vi "ClassList Playground.vi"() -> ()   [LabVIEW 2019]
uses:
  Classes/Subpanel/Edit/Edit/Edit.lvclass
  Classes/Settings/Setting Database/Setting Database.lvclass
  C:/Program Files (x86)/National Instruments/LabVIEW 2019/vi.lib/JKI/JKI SMO/SMO/SMO.lvclass
  Classes/Settings/Setting Database/Typedefs/PrivateEvents--Setting Database.Refresh.ctl
  Classes/Settings/Setting Database/Typedefs/PrivateEvents--Setting Database.SetActivePath.ctl
  Classes/Settings/Setting Database/Typedefs/PrivateEvents--Setting Database.Add To Group.ctl
  Classes/Settings/Setting Database/Typedefs/PrivateEvents--Setting Database.SetActiveRectangle.ctl
  Classes/Subpanel/Manager/Subpanel.Edit.lvclass
  C:/Users/Albro/Documents/GitHub/AFM-Lithography/lvsrc/Classes/Subpanel/Subpanel.lvclass
  Classes/Subpanel/Edit/Edit.Path/Edit.Path.lvclass
  <vilib>/JKI/JKI SMO/SMO/SMO.lvclass
  Classes/Subpanel/Subpanel.lvclass
  C:/Users/Albro/Documents/GitHub/AFM-Lithography/lvsrc/Classes/Subpanel/Edit/Edit/Edit.lvclass
panel:
  out "Array":T1(array[cluster])
  in  "Key":string="p"
  out "key not found?":bool
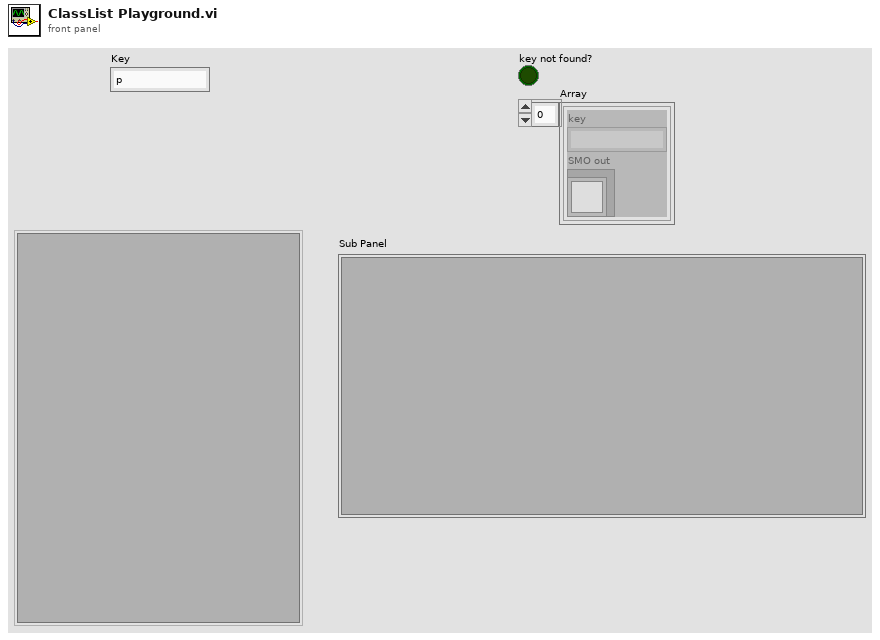
[diagram p1: front panel]
types:
  T1 = cluster{"key":string, "SMO out":refnum<class "Edit.lvclass">}[]
  T2 = typedef "Setting Database.lvclass/PrivateEvents--Setting Database.SetActiveRectangle.ctl" = i32
  T3 = typedef "Setting Database.lvclass/PrivateEvents--Setting Database.Add To Group.ctl" = cluster{"Name":string, "Group":string}
  T4 = typedef "Setting Database.lvclass/PrivateEvents--Setting Database.SetActivePath.ctl" = i32
  T5 = typedef "Setting Database.lvclass/PrivateEvents--Setting Database.Refresh.ctl" = cluster{"Paths":string[], "Rectangles":string[], "Funnels":string[], "Dots":string[]}
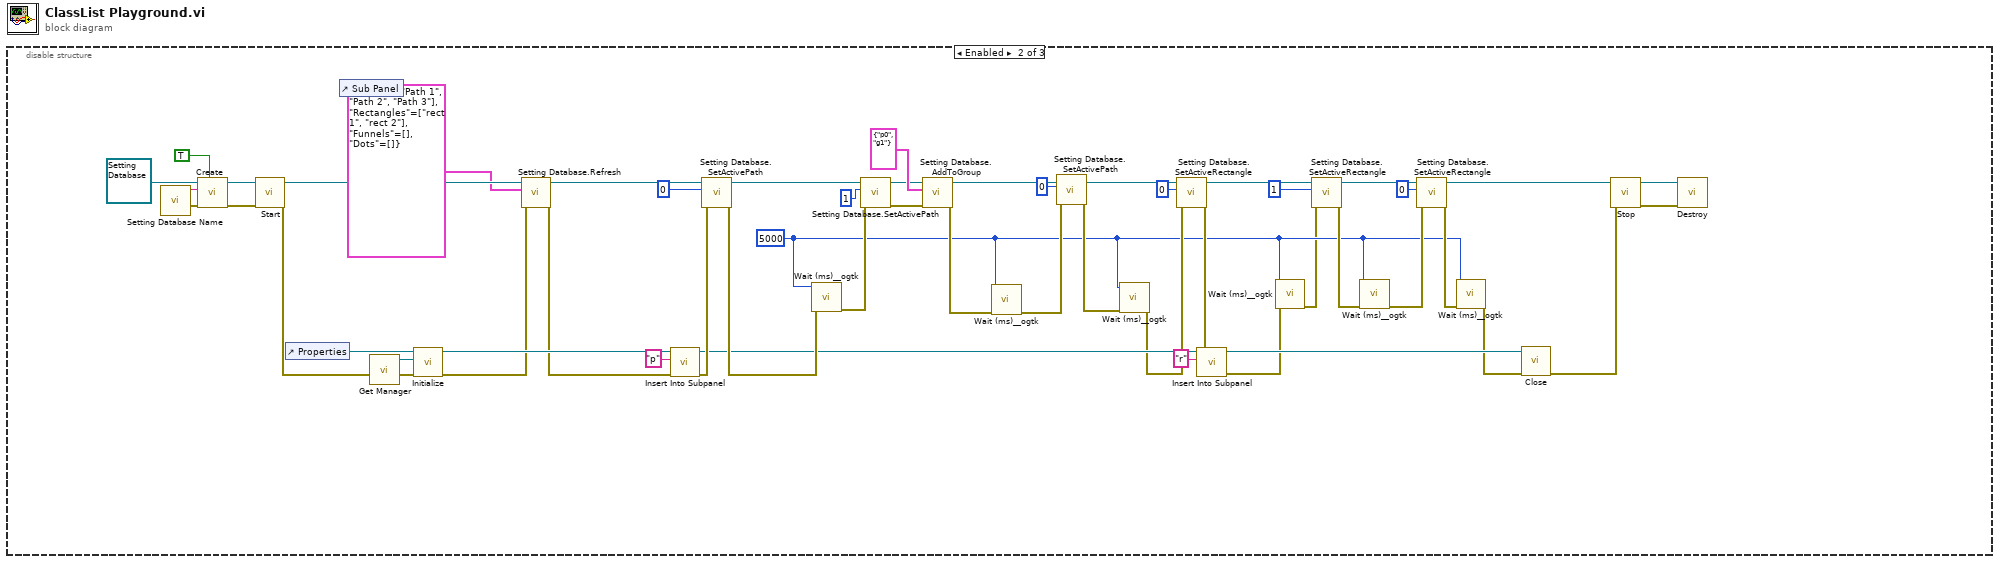
[diagram p0: block diagram]
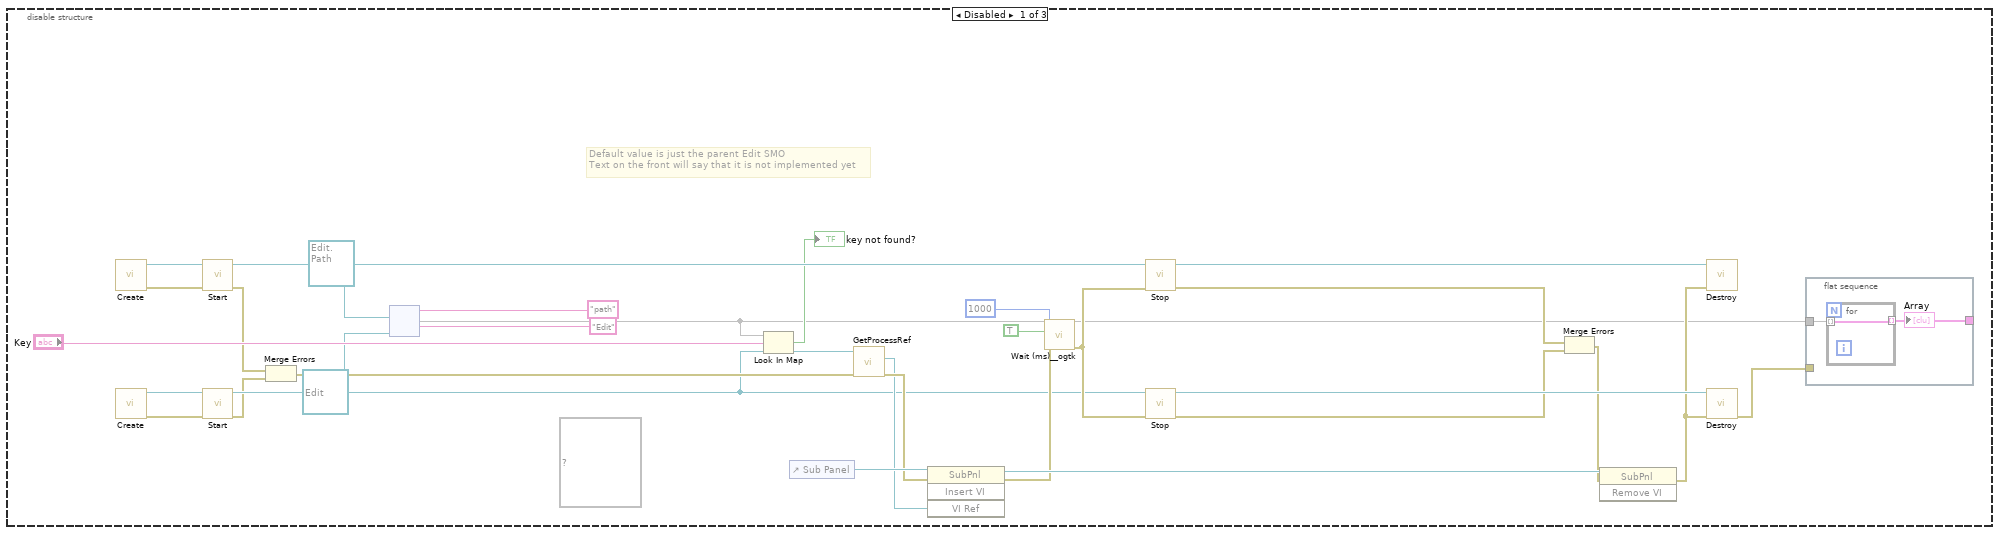
[diagram p2: hidden frame]
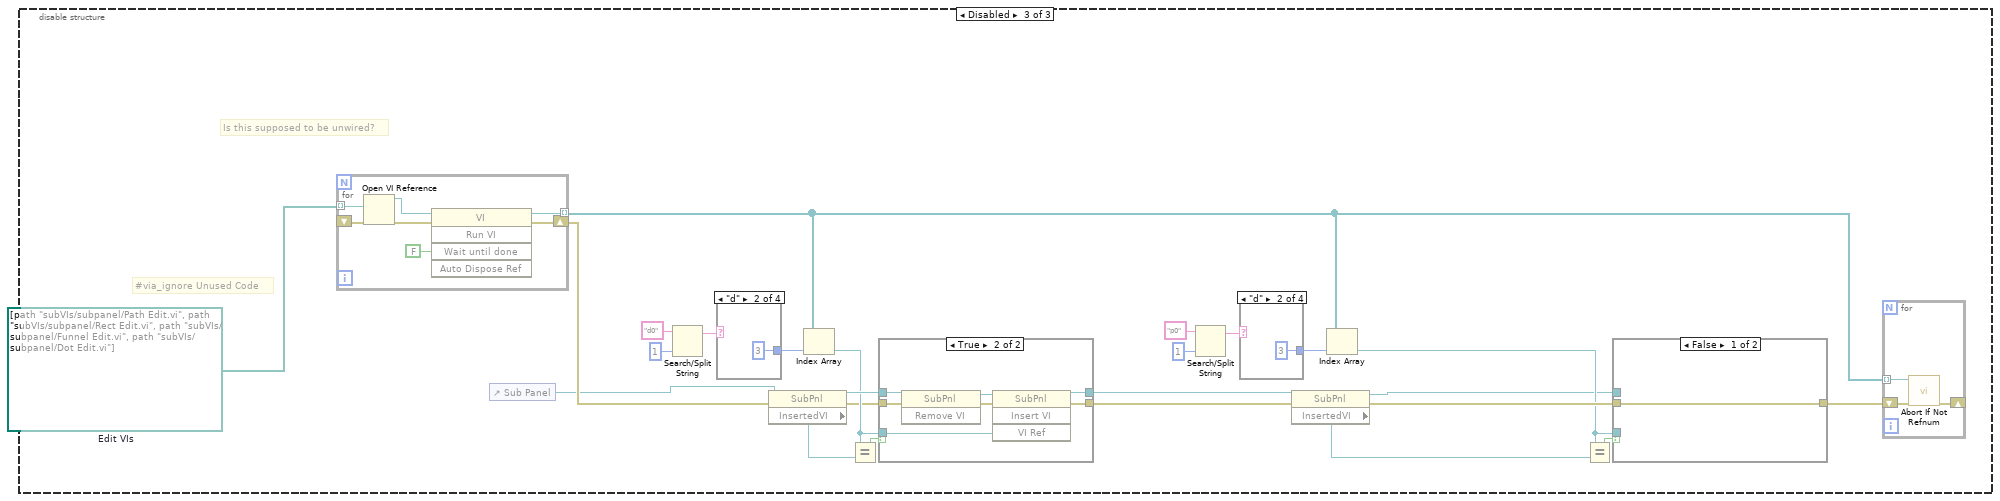
[diagram p3: hidden frame]
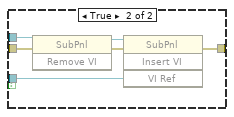
[diagram p4: hidden frame]
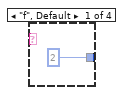
[diagram p5: hidden frame]
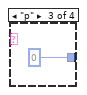
[diagram p6: hidden frame]
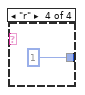
[diagram p7: hidden frame]
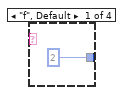
[diagram p9: hidden frame]
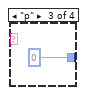
[diagram p10: hidden frame]
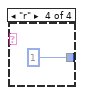
[diagram p11: hidden frame]
diagram:
  n1 = disable-structure shown="Enabled" {
    frame Disabled {
      (unwired) map{string, refnum<class "Edit.lvclass">} {} ("map")
      # "Default value is just the parent Edit SMO\nText on the front will say that it is not implemented yet"
      n2 = call <vilib>:"Create.vi"("SMO"=refnum<class "Edit.Path.lvclass"> refnum ("Edit.Path.lvclass")) -> ("error out"=w16:errorcluster, "SMO out"=w29:refnum<class "Edit.Path.lvclass">)  [unwired: 8 in, 1 out]
      n3 = call <vilib>:"Create.vi"("SMO"=refnum<class "Edit.lvclass"> refnum ("Edit.lvclass")) -> ("error out"=w12:errorcluster, "SMO out"=w30:refnum<class "Edit.lvclass">)  [unwired: 8 in, 1 out]
      n4 = call <vilib>:"Start.vi"("error in (no error)"=w16, "SMO"=w29) -> ("error out"=w15:errorcluster, "SMO out"=w24:refnum<class "Edit.Path.lvclass">)  [unwired: 8 in]
      n5 = call <vilib>:"Start.vi"("error in (no error)"=w12, "SMO"=w30) -> ("error out"=w14:errorcluster, "SMO out"=w3:refnum<class "Edit.lvclass">)  [unwired: 8 in]
      n6 = Merge Errors(w15, w14) -> (w13:errorcluster)
      n7 = node("path" ("key"), w24, "Edit" ("key"), w3) -> (w1:map{string, refnum<class "Edit.lvclass">})
      n8 = Look In Map(map=w1, key="Key", default value=w3) -> (key not found?=→"key not found?":bool, value=w26:refnum<class "Edit.lvclass">)
      n9 = control-ref of="Sub Panel"() -> (w10:refnum<vi>)
      n10 = call "GetProcessRef.vi"("error in (no error)"=w13, "Edit in"=w26) -> ("error out"=w6:errorcluster, "Static VI Ref"=w5:refnum<vi>)  [unwired: 7 in, 1 out]
      n11 = invoke class="SubPnl" method="Insert VI"(reference=w10, error in=w6, "VI Ref"=w5) -> (reference out=w23:refnum<vi>, error out=w7:errorcluster)  [unwired: 1 in, 2 out]
      n12 = call <userlib>:"Wait (ms)__ogtk.vi"("error in (no error)"=w7, "Wait on Error (FALSE)"=TRUE, "milliseconds to wait"=u32 1000) -> ("error out"=w25:errorcluster)  [unwired: 7 in, 1 out]
      n13 = call <vilib>:"Stop.vi"("error in (no error)"=w25, "SMO"=w24) -> ("error out"=w8:errorcluster, "SMO out"=w21:refnum<class "Edit.Path.lvclass">)  [unwired: 8 in]
      n14 = call <vilib>:"Stop.vi"("error in (no error)"=w25, "SMO"=w3) -> ("error out"=w18:errorcluster, "SMO out"=w22:refnum<class "Edit.lvclass">)  [unwired: 8 in]
      n15 = Merge Errors(w8, w18) -> (w19:errorcluster)
      n16 = invoke class="SubPnl" method="Remove VI"(reference=w23, error in=w19) -> (error out=w17:errorcluster)  [unwired: 1 in, 2 out]
      n17 = call <vilib>:"Destroy.vi"("error in (no error)"=w17, "SMO"=w21) -> ()  [unwired: 9 in, 1 out]
      n18 = call <vilib>:"Destroy.vi"("error in (no error)"=w17, "SMO"=w22) -> ("error out"=w2:errorcluster)  [unwired: 9 in]
      n19 = flat-sequence {
        tunnel: w1 -> [w34]
        tunnel: w2 -> [_]
        tunnel: [w33] -> _
        frame #0 {
          n20 = for {
            tunnel: w34 -> [w35] mode=indexing
            tunnel: [w35] -> w33 mode=indexing
          }
          "Array" <- w33
        }
      }
    }
    frame Enabled {
      w41 = u32 5000 ("milliseconds to wait")
      n21 = call "Setting Database Name.vi"() -> ("error out"=w77:errorcluster, "Name"=w78:string)  [unwired: 10 in]
      n22 = call <vilib>:"Create.vi"("Shared Resource (F)"=TRUE, "error in (no error)"=w77, "Subsystem Name (optional)"=w78, "SMO"=refnum<class "Setting Database.lvclass"> refnum ("Setting Database.lvclass")) -> ("error out"=w81:errorcluster, "SMO out"=w82:refnum<class "Setting Database.lvclass">)  [unwired: 5 in, 1 out]
      n23 = call <vilib>:"Start.vi"("error in (no error)"=w81, "SMO"=w82) -> ("error out"=w76:errorcluster, "SMO out"=w72:refnum<class "Setting Database.lvclass">)  [unwired: 8 in]
      n24 = control-ref of="Properties"() -> (w73:refnum<vi>)
      n25 = control-ref of="Sub Panel"() -> ()  [unwired: 1 out]
      n26 = call "Get Manager.vi"("error in (no error)"=w76) -> ("error out"=w75:errorcluster, "Subpanel.Edit"=w74:refnum<class "Subpanel.Edit.lvclass">)  [unwired: 9 in]
      n27 = call "Initialize.vi"("error in (no error)"=w75, "Subpanel.lvclass"=w74, "Sub Panel"=w73) -> ("error out"=w61:errorcluster, "Subpanel out"=w87:refnum<class "Subpanel.Edit.lvclass">)  [unwired: 7 in]
      n28 = call "Setting Database.Refresh.vi"("error in (no error)"=w61, "Initialize"=T5 {"Paths"=["Path 1", "Path 2", "Path 3"], "Rectangles"=["rect 1", "rect 2"], "Funnels"=[], "Dots"=[]}, "Setting Database"=w72) -> ("error out"=w60:errorcluster, "Setting Database out"=w69:refnum<class "Setting Database.lvclass">)  [unwired: 7 in]
      n29 = call "Insert Into Subpanel.vi"("error in (no error)"=w60, "Key"="p", "Subpanel.lvclass"=w87) -> ("error out"=w59:errorcluster, "Subpanel out"=w53:refnum<class "Subpanel.Edit.lvclass">)  [unwired: 7 in]
      n30 = call "Setting Database.SetActivePath.vi"("error in (no error)"=w59, "SetActivePath"=T4 0, "Setting Database"=w69) -> ("error out"=w65:errorcluster, "Setting Database out"=w67:refnum<class "Setting Database.lvclass">)  [unwired: 7 in]
      n31 = call <userlib>:"Wait (ms)__ogtk.vi"("error in (no error)"=w65, "milliseconds to wait"=w41) -> ("error out"=w64:errorcluster)  [unwired: 8 in, 1 out]
      n32 = call "Setting Database.SetActivePath.vi"("error in (no error)"=w64, "SetActivePath"=T4 1, "Setting Database"=w67) -> ("error out"=w56:errorcluster, "Setting Database out"=w57:refnum<class "Setting Database.lvclass">)  [unwired: 7 in]
      n33 = call "Setting Database.AddToGroup.vi"("error in (no error)"=w56, "Add To Group"=T3 {"Name"="p0", "Group"="g1"}, "Setting Database"=w57) -> ("error out"=w55:errorcluster, "Setting Database out"=w51:refnum<class "Setting Database.lvclass">)  [unwired: 7 in]
      n34 = call <userlib>:"Wait (ms)__ogtk.vi"("error in (no error)"=w55, "milliseconds to wait"=w41) -> ("error out"=w62:errorcluster)  [unwired: 8 in, 1 out]
      n35 = call "Setting Database.SetActivePath.vi"("error in (no error)"=w62, "SetActivePath"=T4 0, "Setting Database"=w51) -> ("error out"=w63:errorcluster)  [unwired: 7 in, 1 out]
      n36 = call <userlib>:"Wait (ms)__ogtk.vi"("error in (no error)"=w63, "milliseconds to wait"=w41) -> ("error out"=w48:errorcluster)  [unwired: 8 in, 1 out]
      n37 = call "Setting Database.SetActiveRectangle.vi"("error in (no error)"=w48, "SetActiveRectangle"=T2 0, "Setting Database"=w51) -> ("error out"=w47:errorcluster, "Setting Database out"=w39:refnum<class "Setting Database.lvclass">)  [unwired: 7 in]
      n38 = call "Insert Into Subpanel.vi"("error in (no error)"=w47, "Key"="r", "Subpanel.lvclass"=w53) -> ("error out"=w49:errorcluster, "Subpanel out"=w52:refnum<class "Subpanel.Edit.lvclass">)  [unwired: 7 in]
      n39 = call <userlib>:"Wait (ms)__ogtk.vi"("error in (no error)"=w49, "milliseconds to wait"=w41) -> ("error out"=w37:errorcluster)  [unwired: 8 in, 1 out]
      n40 = call "Setting Database.SetActiveRectangle.vi"("error in (no error)"=w37, "SetActiveRectangle"=T2 1, "Setting Database"=w39) -> ("error out"=w45:errorcluster, "Setting Database out"=w40:refnum<class "Setting Database.lvclass">)  [unwired: 7 in]
      n41 = call <userlib>:"Wait (ms)__ogtk.vi"("error in (no error)"=w45, "milliseconds to wait"=w41) -> ("error out"=w43:errorcluster)  [unwired: 8 in, 1 out]
      n42 = call "Setting Database.SetActiveRectangle.vi"("error in (no error)"=w43, "SetActiveRectangle"=T2 0, "Setting Database"=w40) -> ("error out"=w42:errorcluster, "Setting Database out"=w38:refnum<class "Setting Database.lvclass">)  [unwired: 7 in]
      n43 = call <userlib>:"Wait (ms)__ogtk.vi"("error in (no error)"=w42, "milliseconds to wait"=w41) -> ("error out"=w36:errorcluster)  [unwired: 8 in, 1 out]
      n44 = call "Close.vi"("error in (no error)"=w36, "Subpanel.lvclass"=w52) -> ("error out"=w85:errorcluster)  [unwired: 8 in, 1 out]
      n45 = call <vilib>:"Stop.vi"("error in (no error)"=w85, "SMO"=w38) -> ("error out"=w84:errorcluster, "SMO out"=w83:refnum<class "Setting Database.lvclass">)  [unwired: 8 in]
      n46 = call <vilib>:"Destroy.vi"("error in (no error)"=w84, "SMO"=w83) -> ()  [unwired: 9 in, 1 out]
    }
    frame Disabled {
      w112 = path[] [path "subVIs/subpanel/Path Edit.vi", path "subVIs/subpanel/Rect Edit.vi", path "subVIs/subpanel/Funnel Edit.vi", path "subVIs/subpanel/Dot Edit.vi"]  # Edit VIs
      # "#via_ignore Unused Code"
      # "Is this supposed to be unwired?"
      n47 = for {
        tunnel: [w141] -> w88 mode=indexing
        shift-right: [w144] -> w107
        shift-left: _ -> [w145]
        tunnel: w112 -> [w140] mode=indexing
        # "Load and run Plugin VIs"
        n48 = Open VI Reference(vi path=w140, error in (no error)=w145) -> (vi reference=w142:refnum<vi>, error out=w146:errorcluster)  [unwired: 4 in]
        n49 = invoke on="Invoke Node" class="VI" method="Run VI"(reference=w142, error in=w146, "Wait until done"=FALSE ("Wait Until Done")) -> (reference out=w141:refnum<vi>, error out=w144:errorcluster)  [unwired: 2 in, 3 out]
      }
      n50 = control-ref of="Sub Panel"() -> (w101:refnum<vi>)
      n51 = Search/Split String(string="d0", offset (0)=1) -> (substring before match=w110:string)  [unwired: 1 in, 2 out]
      n52 = case shown="\"d\"" w110 {
        tunnel: [2 3 0 1] -> w111
        frame "f", Default {
        }
        frame "d" {
        }
        frame "p" {
        }
        frame "r" {
        }
      }
      n53 = property class="SubPnl"(reference=w101, error in=w107) -> (reference out=w105:refnum<vi>, error out=w103:errorcluster, "InsertedVI"=w108:refnum<vi>)
      n54 = Index Array(array=w88, index=w111) -> (element=w104:refnum<vi>)
      n55 = Equal?(x=w104, y=w108) -> (x = y?=w106:bool)
      n56 = case shown="True" w106 {
        tunnel: w105 -> [w127 w133]
        tunnel: w104 -> [_ w132]
        tunnel: w103 -> [w128 w131]
        tunnel: [w128 w130] -> w91
        tunnel: [w127 w129] -> w90
        frame False {
        }
        frame True {
          n57 = invoke on="Invoke Node" class="SubPnl" method="Remove VI"(reference=w133, error in=w131) -> (reference out=w134:refnum<vi>, error out=w135:errorcluster)  [unwired: 1 in, 1 out]
          n58 = invoke on="Invoke Node" class="SubPnl" method="Insert VI"(reference=w134, error in=w135, "VI Ref"=w132) -> (reference out=w129:refnum<vi>, error out=w130:errorcluster)  [unwired: 1 in, 2 out]
        }
      }
      n59 = Search/Split String(string="p0", offset (0)=1) -> (substring before match=w93:string)  [unwired: 1 in, 2 out]
      n60 = case shown="\"d\"" w93 {
        tunnel: [2 3 0 1] -> w92
        frame "f", Default {
        }
        frame "d" {
        }
        frame "p" {
        }
        frame "r" {
        }
      }
      n61 = property class="SubPnl"(reference=w90, error in=w91) -> (reference out=w97:refnum<vi>, error out=w99:errorcluster, "InsertedVI"=w95:refnum<vi>)
      n62 = Index Array(array=w88, index=w92) -> (element=w98:refnum<vi>)
      n63 = Equal?(x=w98, y=w95) -> (x = y?=w96:bool)
      n64 = case shown="False" w96 {
        tunnel: w97 -> [_ w120]
        tunnel: w98 -> [_ w119]
        tunnel: w99 -> [w116 w118]
        tunnel: [w116 w117] -> w89
        frame False {
        }
        frame True {
          n65 = invoke on="Invoke Node" class="SubPnl" method="Remove VI"(reference=w120, error in=w118) -> (reference out=w121:refnum<vi>, error out=w122:errorcluster)  [unwired: 1 in, 1 out]
          n66 = invoke on="Invoke Node" class="SubPnl" method="Insert VI"(reference=w121, error in=w122, "VI Ref"=w119) -> (error out=w117:errorcluster)  [unwired: 1 in, 3 out]
        }
      }
      n67 = for {
        tunnel: w88 -> [w113] mode=indexing
        shift-right: [w114] -> _
        shift-left: w89 -> [w115]
        n68 = call "Abort If Not Refnum.vi"("error in (no error)"=w115, "VI in"=w113) -> ("error out"=w114:errorcluster)  [unwired: 9 in]
      }
    }
  }
